vi "to string.vi"(8 "error in":errorcluster, 11 "SQLite configuration in":refnum<class "SQLite configuration.lvclass">) -> (0 "error out":errorcluster, 1 "data":string, 2 "version":string, 3 "SQLite configuration out":refnum<class "SQLite configuration.lvclass">)   [LabVIEW 2014, in "SQLite configuration.lvclass"]
doc: "Provides an interface for saving a module configuration to a file or other serialized data source. It is recommended that all children of this class store data in two sets--data required for its own initialization, and any data required for parent initialization--and that each implementation uses the <b>Call Parent Method</b> primitive to serialize parent information."
uses:
  SQLite configuration.lvclass
  SQLite configuration.lvclass/SQLite configuration.ctl
  current version.vi
  <vilib>/NI/Tag Bus Module Framework/module configuration/TBM module configuration.lvclass
  <vilib>/NI/Tag Bus Module Framework/channel/TBM channel.lvclass
  <vilib>/NI/Configuration Framework/serializable configuration/NISE_CEF_serializable configuration.lvclass
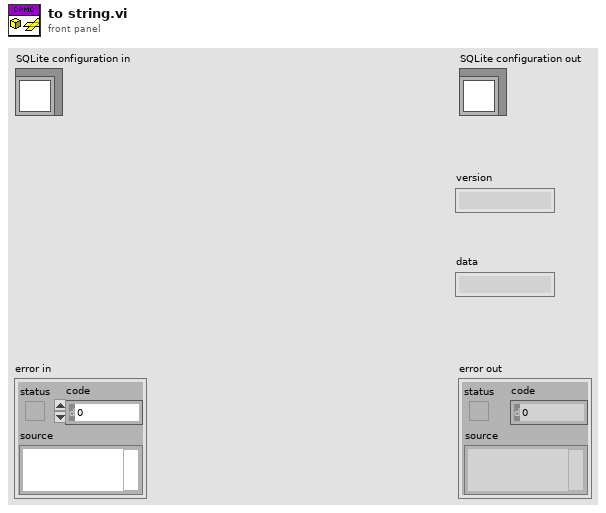
[diagram p1: front panel]
types:
  T1 = typedef "SQLite configuration.lvclass/Line.ctl" = cluster{"channel":refnum<class "TBM channel.lvclass">}
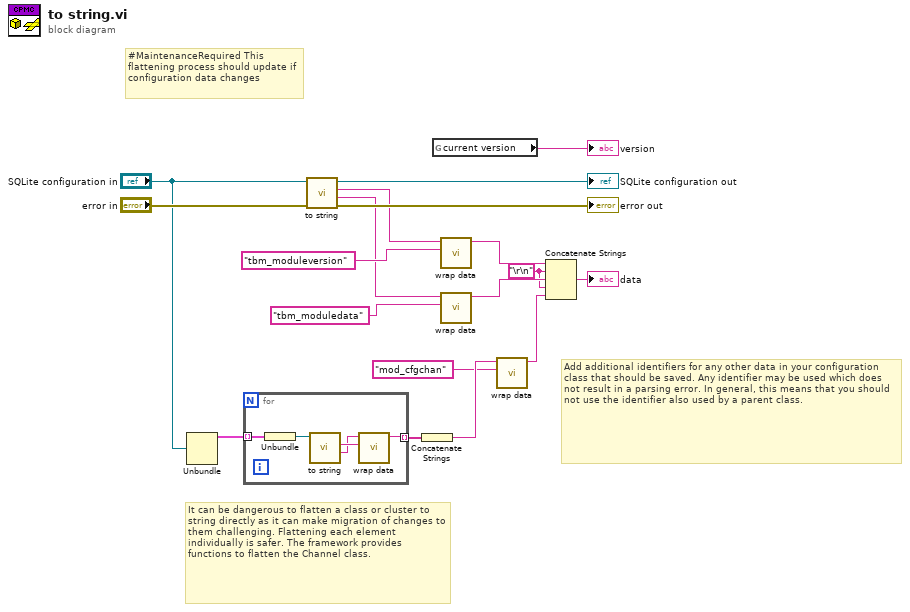
[diagram p0: block diagram]
diagram:
  w5 = "\r\n"
  # "It can be dangerous to flatten a class or cluster to string directly as it can make migration of changes to them challenging. Flattening each element individually is safer. The framework provides functions to flatten the Channel class."
  # "Add additional identifiers for any other data in your configuration class that should be saved. Any identifier may be used which does not result in a parsing error. In general, this means that you should not use the identifier also used by a parent class."
  # "#MaintenanceRequired This flattening process should update if configuration data changes"
  n1 = Unbundle("SQLite configuration in") -> (w4:T1[])  [unwired: 3 out]
  n2 = for {
    tunnel: w4 -> [w23] mode=indexing
    tunnel: [w19] -> w3 mode=indexing
    n3 = Unbundle(w23) -> ("channel"=w22:refnum<class "TBM channel.lvclass">)
    n4 = call-dynamic "to string.vi"("channel in"=w22) -> ("channel data"=w20:string, "identifier"=w21:string)  [unwired: 7 in, 2 out]
    n5 = call <vilib>:"wrap data.vi"("identifier"=w21, "data to wrap"=w20) -> ("wrapped data"=w19:string)  [unwired: 9 in]
  }
  n6 = call-parent "to string.vi"("error in"="error in", "module configuration in"="SQLite configuration in") -> ("error out"=→"error out":errorcluster, "data"=w9:string, "version"=w10:string, "module configuration out"=→"SQLite configuration out":refnum<class "SQLite configuration.lvclass">)  [unwired: 6 in]
  n7 = Concatenate Strings(w3) -> (w2:string)
  n8 = global read "current version.vi" "current version"() -> (→"version":string)
  n9 = call <vilib>:"wrap data.vi"("identifier"="tbm_moduleversion" ("additional identifier"), "data to wrap"=w10) -> ("wrapped data"=w12:string)  [unwired: 9 in]
  n10 = call <vilib>:"wrap data.vi"("identifier"="tbm_moduledata" ("additional identifier"), "data to wrap"=w9) -> ("wrapped data"=w11:string)  [unwired: 9 in]
  n11 = call <vilib>:"wrap data.vi"("identifier"="mod_cfgchan", "data to wrap"=w2) -> ("wrapped data"=w6:string)  [unwired: 9 in]
  n12 = Concatenate Strings(w12, w5, w11, w5, w6) -> (→"data":string)
